vi "Demo.vi"() -> ()   [LabVIEW 2012, in "Mlistbox Tools.lvlib"]
uses:
  Mlistbox Tools.lvlib
  ListBox/Custom Type/Read and Write Mode.ctl
  Custom Type/Row and Col Option.ctl
  ListBox/Listbox Tool.lvlib
panel:
  in  "多列列表框":i32(listbox)
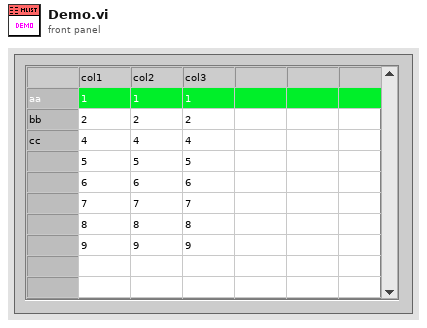
[diagram p1: front panel]
types:
  T1 = typedef "Mlistbox Tools.lvlib/Row and Col Option.ctl" = enum16{"Row", "Col"}
  T2 = typedef "Listbox Tool.lvlib/Read and Write Mode.ctl" = enum16{"Read", "Write"}
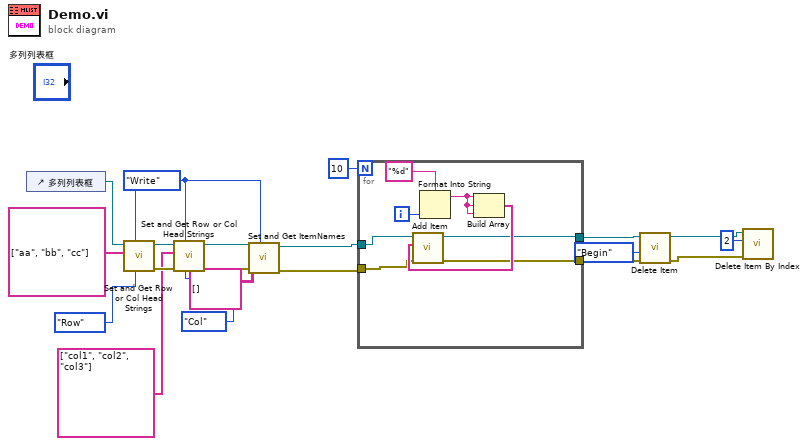
[diagram p0: block diagram]
diagram:
  w5 = Read_and_Write_Mode."Write" ("Mode")
  n1 = control-ref of="多列列表框"() -> (w20:refnum<vi>)
  n2 = call "Set and Get Row or Col Head Strings.vi"("Row Or Col"=Row_and_Col_Option."Row", "Mode"=w5, "String[]  In"=string[] ["aa", "bb", "cc"], "Mlistbox Ref"=w20) -> ("错误输出"=w18:errorcluster, "Mlistbox Ref Dup"=w17:refnum<vi>)  [unwired: 5 in, 1 out]
  n3 = call "Set and Get Row or Col Head Strings.vi"("Row Or Col"=Row_and_Col_Option."Col", "Mode"=w5, "错误输入"=w18, "String[]  In"=string[] ["col1", "col2", "col3"], "Mlistbox Ref"=w17) -> ("错误输出"=w9:errorcluster, "Mlistbox Ref Dup"=w10:refnum<vi>)  [unwired: 4 in, 1 out]
  n4 = call "Set and Get ItemNames.vi"("Mode"=w5, "错误输入"=w9, "ItemNames In"=string[][] [], "Mlistbox Ref"=w10) -> ("错误输出"=w6:errorcluster, "Mlistbox Ref Dup"=w7:refnum<vi>)  [unwired: 5 in, 1 out]
  n5 = for {
    N: 10 -> [_]
    tunnel: w6 -> [w23]
    tunnel: w7 -> [w25]
    tunnel: [w22] -> w11
    tunnel: [w21] -> w12
    i -> [w28]
    n6 = Format Into String(format string="%d" ("格式字符串"), w28) -> (resulting string=w26:string)  [unwired: 2 in, 1 out]
    n7 = Build Array(w26, w26, w26) -> (w24:string[])
    n8 = call "Add Item.vi"("错误输入"=w23, "Item"=w24, "Mlistbox Ref"=w25) -> ("错误输出"=w22:errorcluster, "Mlistbox Ref Dup"=w21:refnum<vi>)  [unwired: 7 in]
  }
  n9 = call "Delete Item.vi"("错误输入"=w11, "Mode"=enum16{"End", "Begin"}."Begin", "Mlistbox Ref"=w12) -> ("错误输出"=w2:errorcluster, "Mlistbox Ref Dup"=w3:refnum<vi>)  [unwired: 7 in]
  n10 = call "Delete Item By Index.vi"("错误输入"=w2, "Index"=2, "Mlistbox Ref"=w3) -> ()  [unwired: 7 in, 2 out]
